vi "Write Channels.vi"(11 "HW Inline Ctrl in":T1 {"Input Channels"."Input Block Data Refs"."Data Reference" format="%.0x"; "Output Channels"."Output Block Data Refs"."Data Reference" format="%.0x"}) -> (3 "HW Inline Ctrl out":T1 {"Input Channels"."Input Block Data Refs"."Data Reference" format="%.0x"; "Output Channels"."Output Block Data Refs"."Data Reference" format="%.0x"})   [LabVIEW 2015, in "Shared Variable Custom Device.lvlib"]
doc: "Reads the RT FIFO Write and writes the values to the Output Block Data References to update the Output channels."
uses:
  Shared Variable Custom Device.lvlib
  HW Inline Ctrl.ctl
  <vilib>/NI Veristand/Custom Device API/Block Data Reference.ctl
  <vilib>/NI Veristand/Custom Device API/Data Reference.ctl
  <vilib>/NI Veristand/Custom Device API/Global Data Refs.vi
  <vilib>/NI Veristand/Custom Device API/Custom Device API.lvlib
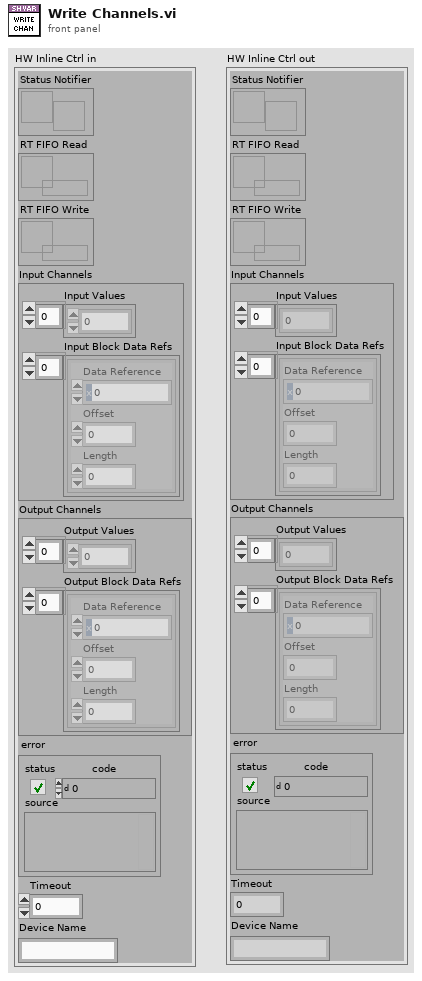
[diagram p1: front panel]
types:
  T1 = typedef "Shared Variable Custom Device.lvlib/HW Inline Ctrl.ctl" = cluster{"Status Notifier":refnum<notifier>, "RT FIFO Read":refnum<k33>, "RT FIFO Write":refnum<k33>, "Input Channels":cluster{"Input Values":dbl[], "Input Block Data Refs":T2[]}, "Output Channels":cluster{"Output Values":dbl[], "Output Block Data Refs":T2[]}, "error":errorcluster, "Timeout":i32, "Device Name":string}
  T2 = typedef "Custom Device API.lvlib/Block Data Reference.ctl" = cluster{"Data Reference":T3, "Offset":u64, "Length":u64}
  T3 = typedef "Custom Device API.lvlib/Data Reference.ctl" = i32
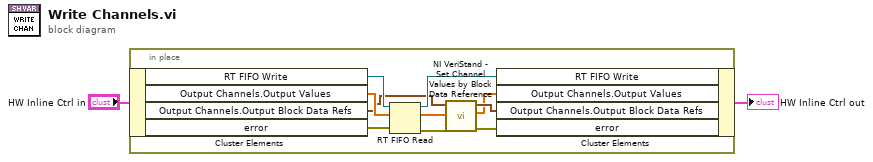
[diagram p0: block diagram]
diagram:
  n1 = in-place {
    n2 = in-place-cluster #1("HW Inline Ctrl in") -> ("RT FIFO Write"=w11:refnum<k33>, "Output Channels.Output Values"=w10:dbl[], "Output Channels.Output Block Data Refs"=w6:T2[], "error"=w12:errorcluster)
    n3 = RT FIFO Read(0:w11, 1:w10, 3:w12) -> (8:w9:refnum<k33>, 9:w7:dbl[], 11:w8:errorcluster)  [unwired: 1 in, 2 out]
    n4 = call <vilib>:"NI VeriStand - Set Channel Values by Block Data Reference.vi"("error in (no error)"=w8, "Values Array in"=w7, "Block Data Ref"=w6) -> ("error out"=w3:errorcluster, "Values Array out"=w4:dbl[], "Block Data Ref dup"=w5:T2[])  [unwired: 6 in]
    n5 = in-place-cluster #1("RT FIFO Write"=w9, "Output Channels.Output Values"=w4, "Output Channels.Output Block Data Refs"=w5, "error"=w3) -> (→"HW Inline Ctrl out":T1)
  }
